vi "Add Data Replay RTM.vi"(8 "error in (no error)":errorcluster, 11 "Node Ptr":u64 format="%.0x") -> (0 "error out":errorcluster)   [LabVIEW 2011, in "Engine Sim System Explorer.lvlib"]
uses:
  Engine Sim System Explorer.lvlib
  Shared/Engine Simulation Global.vi
  <vilib>/NI Veristand/Custom Device API/NI VeriStand - Add Custom Device Section.vi
  <vilib>/NI Veristand/Custom Device API/NI VeriStand - Set Item Property.vi
  <vilib>/NI Veristand/Custom Device API/Set Item Property (Boolean).vi
  <vilib>/Utility/error.llb/Error Cluster From Error Code.vi
  <vilib>/NI Veristand/Custom Device API/NI VeriStand - Add Custom Device Channel.vi
  <vilib>/NI Veristand/Custom Device API/Custom Device API.lvlib
  <vilib>/NI Veristand/Custom Device Tools/Custom Device Utility Library/Custom Device Utility Library.lvlib
panel:
  in  "Tag":string
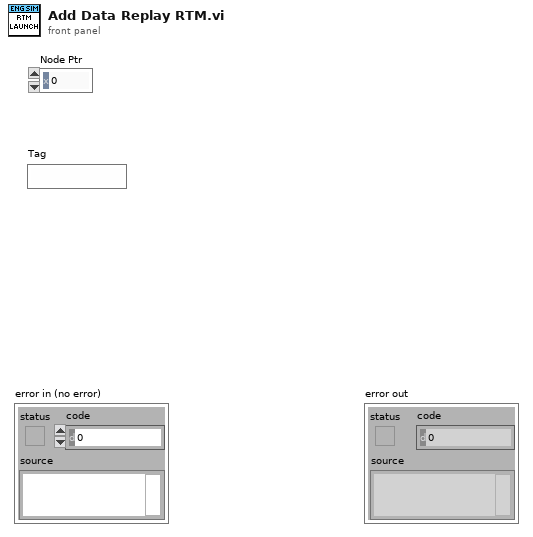
[diagram p1: front panel]
types:
  T1 = typedef "Custom Device API.lvlib/Custom Device Item Info.ctl" = cluster{"Name":string, "Is Channel":bool, "GUID":string}
  T2 = typedef "Custom Device API.lvlib/Custom Device Item Ref.ctl" = u64
  T3 = typedef "Engine Sim System Explorer.lvlib/DataReplayComp.ctl" = cluster{"Name":string, "Number":i32, "Optionals":bool[]}
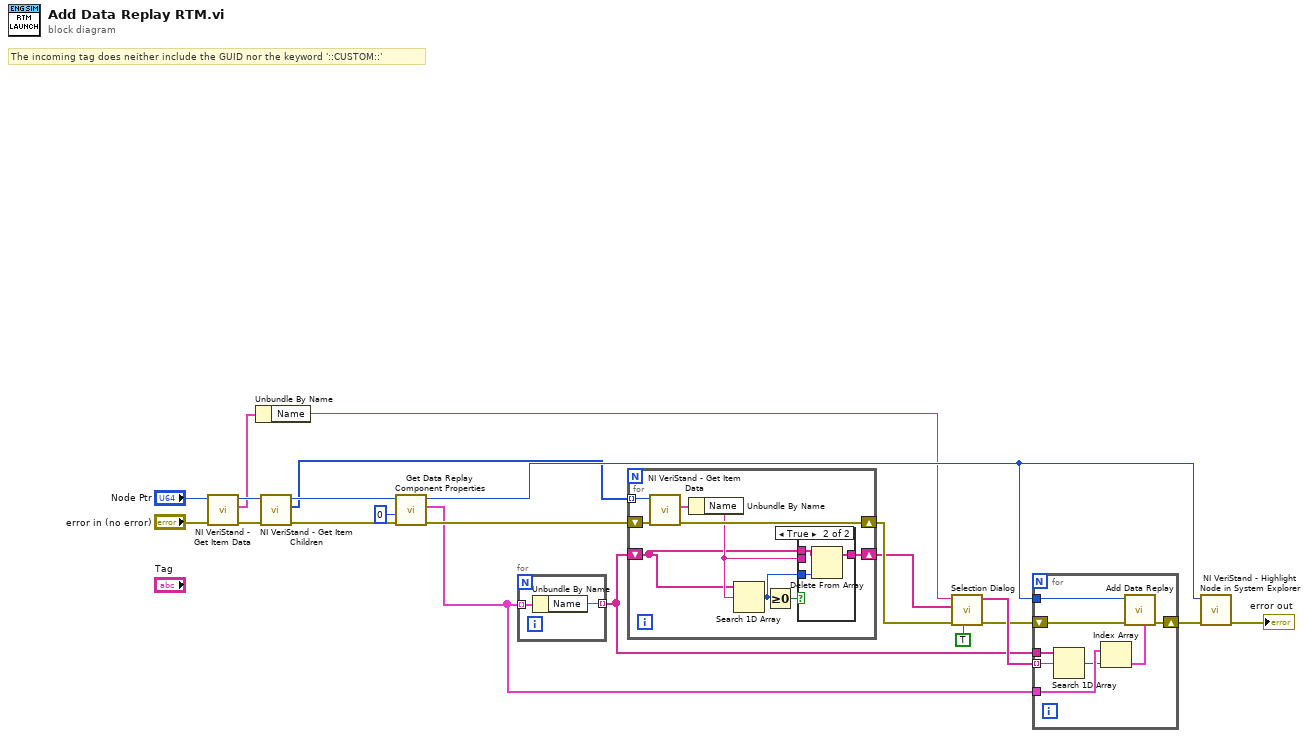
[diagram p0: block diagram]
diagram:
  # "The incoming tag does neither include the GUID nor the keyword '::CUSTOM::'"
  n1 = call <vilib>:"NI VeriStand - Get Item Data.vi"("error in (no error)"="error in (no error)", "Item Ref in"="Node Ptr") -> ("error out"=w10:errorcluster, "Item Info"=w7:T1, "Item Ref out"=w8:T2)  [unwired: 6 in, 1 out]
  n2 = Unbundle By Name(w7) -> ("Name"=w6:string)
  n3 = call <vilib>:"NI VeriStand - Get Item Children.vi"("error in (no error)"=w10, "Item Ref in"=w8) -> ("error out"=w15:errorcluster, "Child Refs"=w16:T2[], "Item Ref out"=w17:T2)  [unwired: 6 in, 1 out]
  n4 = call "Get Data Replay Component Properties.vi"("error in (no error)"=w15, "Prefix #"=0, "Item Ref in"=w17) -> ("error out"=w3:errorcluster, "DataReplays"=w1:T3[], "Item Ref out"=w18:T2)  [unwired: 6 in]
  n5 = for {
    tunnel: w1 -> [w23] mode=indexing
    tunnel: [w22] -> w4 mode=indexing
    n6 = Unbundle By Name(w23) -> ("Name"=w22:string)
  }
  n7 = for {
    tunnel: w16 -> [w32] mode=indexing
    shift-right: [w30] -> w13
    shift-left: w3 -> [w29]
    shift-right: [w27] -> w5
    shift-left: w4 -> [w25]
    n8 = call <vilib>:"NI VeriStand - Get Item Data.vi"("error in (no error)"=w29, "Item Ref in"=w32) -> ("error out"=w30:errorcluster, "Item Info"=w31:T1)  [unwired: 6 in, 2 out]
    n9 = Unbundle By Name(w31) -> ("Name"=w26:string)
    n10 = Search 1D Array(1D array=w25, element=w26) -> (index of element=w24:i32)  [unwired: 1 in]
    n11 = Greater Or Equal To 0?(x=w24) -> (x >= 0?=w28:bool)
    n12 = case shown="True" w28 {
      tunnel: [w33 w35] -> w27
      tunnel: w26 -> [_ _]
      tunnel: w25 -> [w33 w36]
      tunnel: w24 -> [_ w34]
      frame False {
      }
      frame True {
        n13 = Delete From Array(array=w36, index=w34) -> (array with subset deleted=w35:string[])  [unwired: 1 in, 1 out]
      }
    }
  }
  n14 = call "Selection Dialog.vi"("Multi-Selection?"=TRUE, "error in (no error)"=w13, "Tree Items"=w5, "Root Tag"=w6) -> ("error out"=w11:errorcluster, "Selected Names"=w12:string[])  [unwired: 5 in, 1 out]
  n15 = for {
    tunnel: w12 -> [w44] mode=indexing
    shift-right: [w37] -> w20
    shift-left: w11 -> [w40]
    tunnel: w4 -> [w43]
    tunnel: w1 -> [w42]
    tunnel: w18 -> [w38]
    n16 = Search 1D Array(1D array=w43, element=w44) -> (index of element=w41:i32)  [unwired: 1 in]
    n17 = Index Array(array=w42, index=w41) -> (element=w39:T3)
    n18 = call "Add Data Replay.vi"("DataReplay"=w39, "error in (no error)"=w40, "Section Ptr"=w38) -> ("error out"=w37:errorcluster)  [unwired: 8 in]
  }
  n19 = call <vilib>:"NI VeriStand - Highlight Node in System Explorer.vi"("error in (no error)"=w20, "Item Ref in"=w18) -> ("error out"=→"error out":errorcluster)  [unwired: 8 in, 1 out]
